vi "PS_CMD.vi"(4 "?":T1=enum."Cond_EIS", 5 "MSP_I-Range":string="C", 6 "wait until completion? (T)":bool=TRUE, 7 "GUID":string) -> (1 "File Path Out":path[](array[path]), 3 "Enum":T1=enum."Cond_EIS")   [LabVIEW 2019]
uses:
  5_Controls/PS_CMD_type-def.ctl
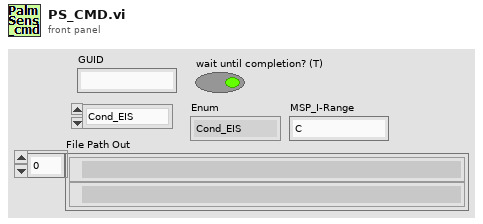
[diagram p1: front panel]
types:
  T1 = typedef "PS_CMD_type-def.ctl" = enum16{"Cond+Temp", "Cond_EIS", "Temp_EIS", "Vwind_MSP", "LongCond", "Cell1_EIS", "Cell2_EIS", "Cell3_EIS"}
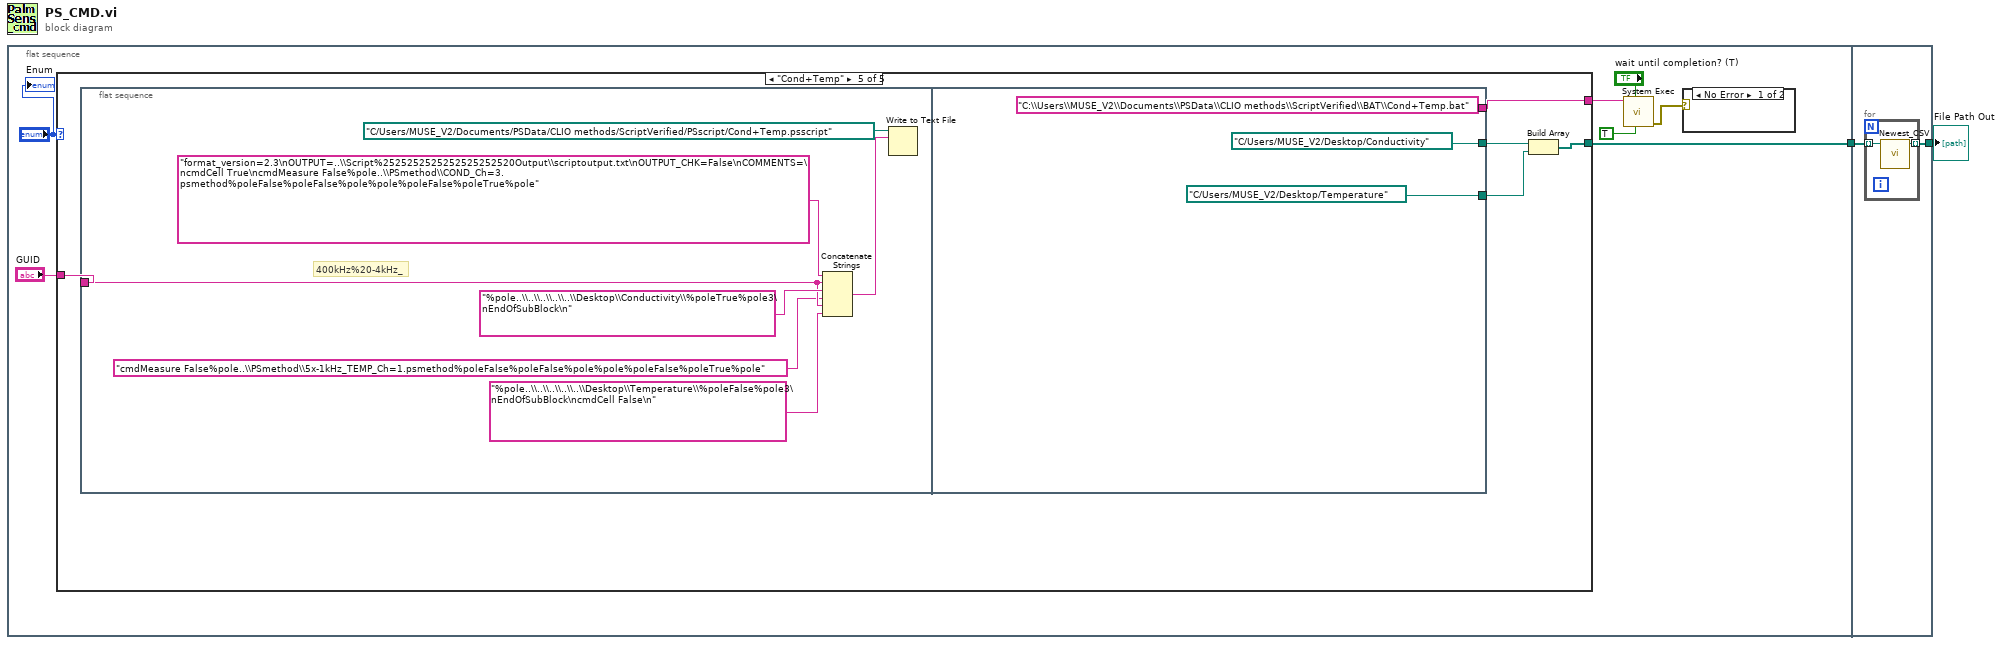
[diagram p0: block diagram]
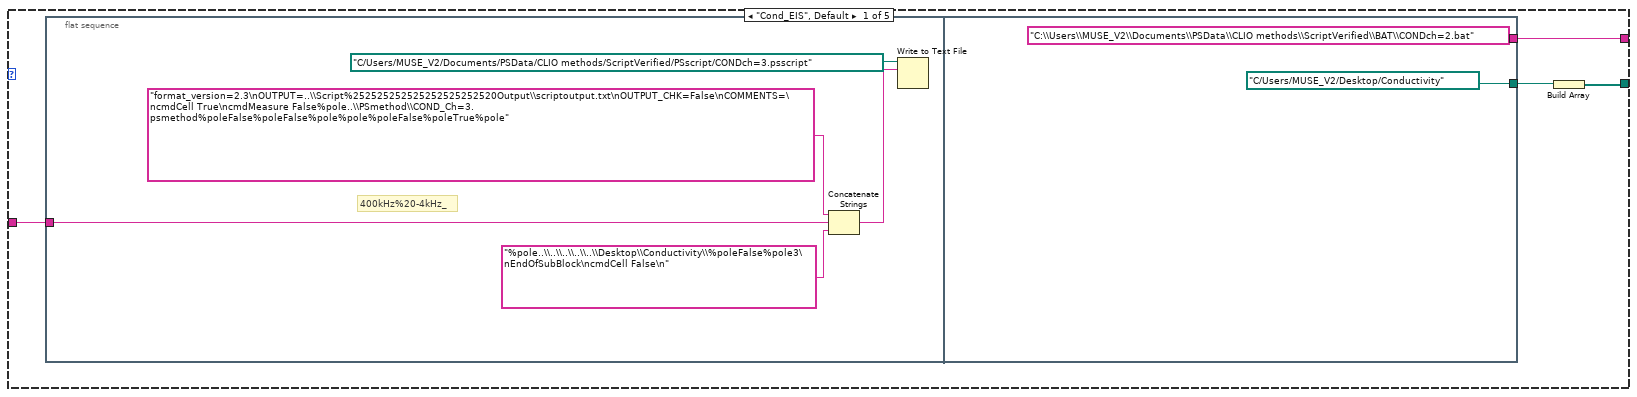
[diagram p3: hidden frame]
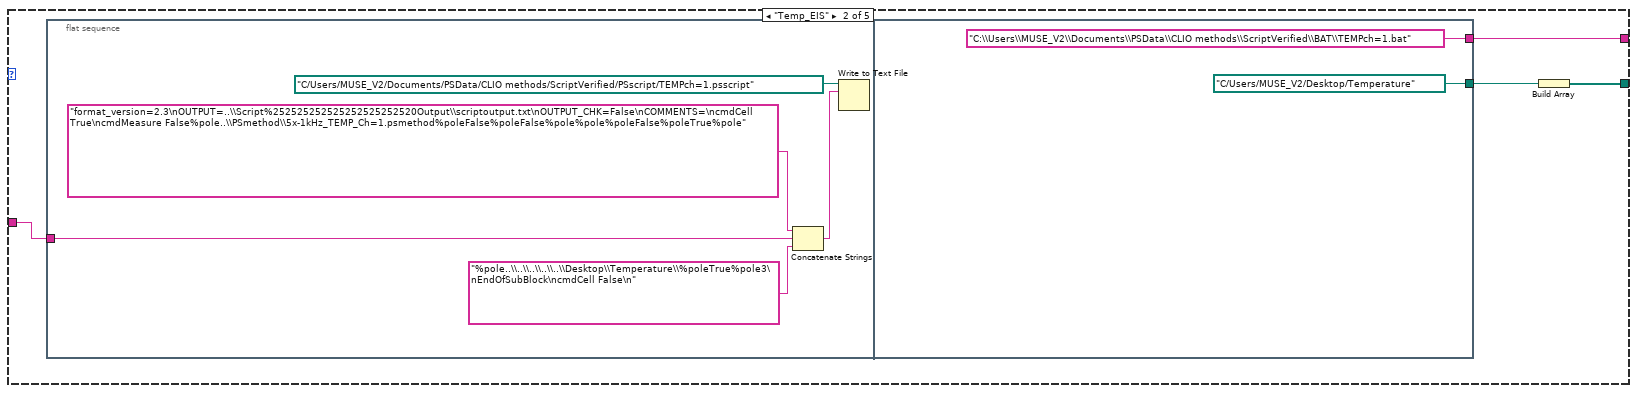
[diagram p4: hidden frame]
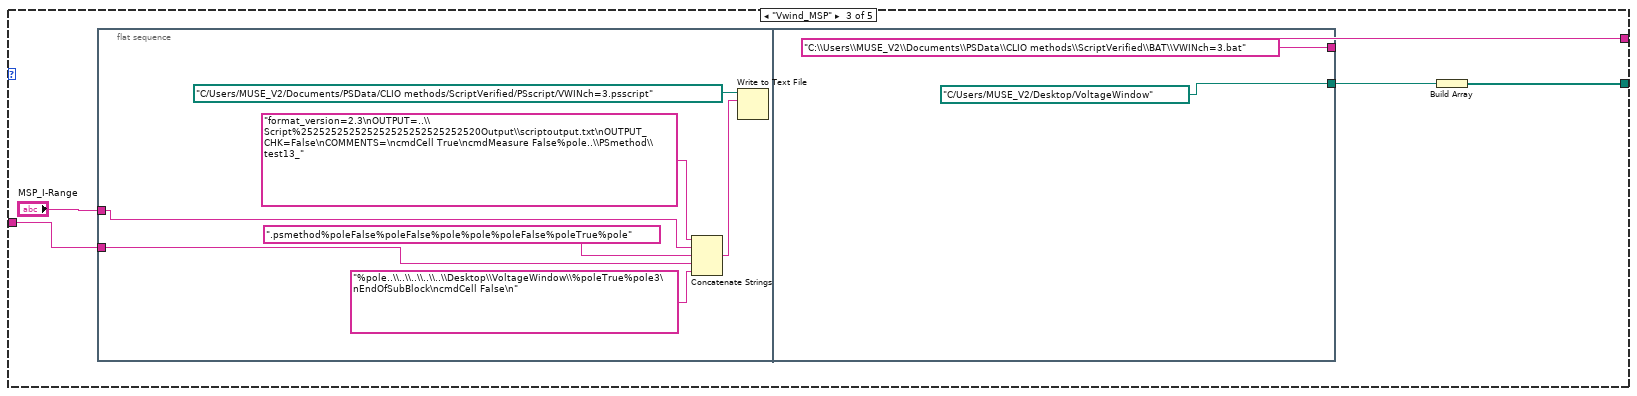
[diagram p5: hidden frame]
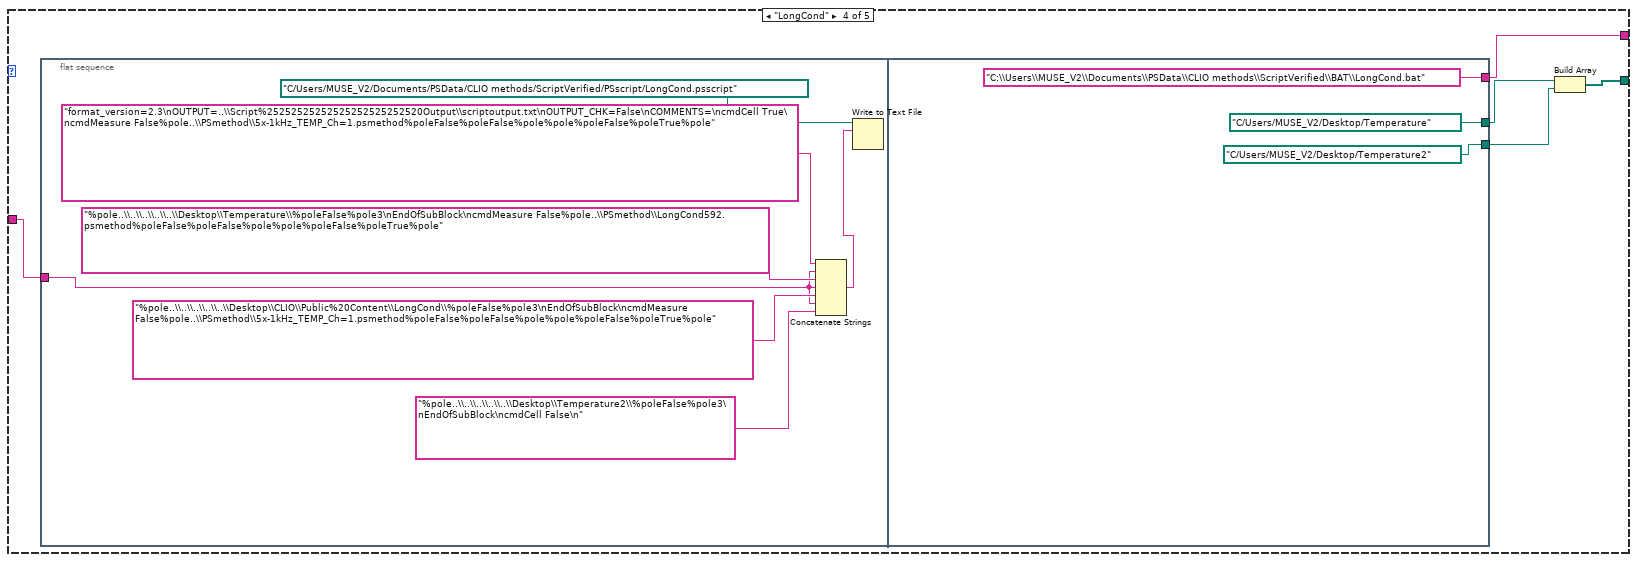
[diagram p6: hidden frame]
diagram:
  n1 = flat-sequence {
    tunnel: [w6] -> w2
    tunnel: w2 -> [w77]
    tunnel: [w76] -> w1
    frame #0 {
      n2 = case shown="\"Cond+Temp\"" "?" {
        tunnel: [w13 w24 w35 w48 w64] -> w7
        tunnel: [w10 w21 w33 w49 w62] -> w6
        tunnel: "GUID" -> [w12 w23 w36 w47 w65]
        frame "Cond_EIS", Default {
          n3 = flat-sequence {
            tunnel: w12 -> [w14]
            tunnel: ["C:\\Users\\MUSE_V2\\Documents\\PSData\\CLIO methods\\ScriptVerified\\BAT\\CONDch=2.bat" ("command line")] -> w13
            tunnel: [path "C:/Users/MUSE_V2/Desktop/Conductivity" ("Folder Path In")] -> w11
            frame #0 {
              # "400kHz%20-4kHz_"
              n4 = Concatenate Strings("format_version=2.3\nOUTPUT=..\\Script%252525252525252525252520Output\\scriptoutput.txt\nOUTPUT_CHK=False\nCOMMENTS=\ncmdCell True\ncmdMeasure False%pole..\\PSmethod\\COND_Ch=3.psmethod%poleFalse%poleFalse%pole%pole%poleFalse%poleTrue%pole" ("text"), w14, "%pole..\\..\\..\\..\\..\\Desktop\\Conductivity\\%poleFalse%pole3\nEndOfSubBlock\ncmdCell False\n" ("string")) -> (w15:string)
              n5 = Write to Text File(file (use dialog)=path "C:/Users/MUSE_V2/Documents/PSData/CLIO methods/ScriptVerified/PSscript/CONDch=3.psscript", text=w15) -> ()  [unwired: 2 in, 3 out]
            }
            frame #1 {
            }
          }
          n6 = Build Array(w11) -> (w10:path[])
        }
        frame "Temp_EIS" {
          n7 = flat-sequence {
            tunnel: w23 -> [w25]
            tunnel: ["C:\\Users\\MUSE_V2\\Documents\\PSData\\CLIO methods\\ScriptVerified\\BAT\\TEMPch=1.bat" ("command line")] -> w24
            tunnel: [path "C:/Users/MUSE_V2/Desktop/Temperature" ("Folder Path In")] -> w22
            frame #0 {
              n8 = Concatenate Strings("format_version=2.3\nOUTPUT=..\\Script%252525252525252525252520Output\\scriptoutput.txt\nOUTPUT_CHK=False\nCOMMENTS=\ncmdCell True\ncmdMeasure False%pole..\\PSmethod\\5x-1kHz_TEMP_Ch=1.psmethod%poleFalse%poleFalse%pole%pole%poleFalse%poleTrue%pole" ("text"), w25, "%pole..\\..\\..\\..\\..\\Desktop\\Temperature\\%poleTrue%pole3\nEndOfSubBlock\ncmdCell False\n" ("string")) -> (w29:string)
              n9 = Write to Text File(file (use dialog)=path "C:/Users/MUSE_V2/Documents/PSData/CLIO methods/ScriptVerified/PSscript/TEMPch=1.psscript", text=w29) -> ()  [unwired: 2 in, 3 out]
            }
            frame #1 {
            }
          }
          n10 = Build Array(w22) -> (w21:path[])
        }
        frame "Vwind_MSP" {
          n11 = flat-sequence {
            tunnel: w36 -> [w39]
            tunnel: "MSP_I-Range" -> [w37]
            tunnel: ["C:\\Users\\MUSE_V2\\Documents\\PSData\\CLIO methods\\ScriptVerified\\BAT\\VWINch=3.bat" ("command line")] -> w35
            tunnel: [path "C:/Users/MUSE_V2/Desktop/VoltageWindow" ("Folder Path In")] -> w34
            frame #0 {
              n12 = Concatenate Strings("format_version=2.3\nOUTPUT=..\\Script%252525252525252525252525252520Output\\scriptoutput.txt\nOUTPUT_CHK=False\nCOMMENTS=\ncmdCell True\ncmdMeasure False%pole..\\PSmethod\\test13_" ("text"), w37, ".psmethod%poleFalse%poleFalse%pole%pole%poleFalse%poleTrue%pole" ("string"), w39, "%pole..\\..\\..\\..\\..\\Desktop\\VoltageWindow\\%poleTrue%pole3\nEndOfSubBlock\ncmdCell False\n" ("string")) -> (w43:string)
              n13 = Write to Text File(file (use dialog)=path "C:/Users/MUSE_V2/Documents/PSData/CLIO methods/ScriptVerified/PSscript/VWINch=3.psscript", text=w43) -> ()  [unwired: 2 in, 3 out]
            }
            frame #1 {
            }
          }
          n14 = Build Array(w34) -> (w33:path[])
        }
        frame "LongCond" {
          n15 = flat-sequence {
            tunnel: w47 -> [w51]
            tunnel: ["C:\\Users\\MUSE_V2\\Documents\\PSData\\CLIO methods\\ScriptVerified\\BAT\\LongCond.bat" ("command line")] -> w48
            tunnel: [path "C:/Users/MUSE_V2/Desktop/Temperature" ("Folder Path In")] -> w50
            tunnel: [path "C:/Users/MUSE_V2/Desktop/Temperature2" ("Folder Path In")] -> w46
            frame #0 {
              # "400kHz%20-4kHz_"
              n16 = Concatenate Strings("format_version=2.3\nOUTPUT=..\\Script%25252525252525252525252520Output\\scriptoutput.txt\nOUTPUT_CHK=False\nCOMMENTS=\ncmdCell True\ncmdMeasure False%pole..\\PSmethod\\5x-1kHz_TEMP_Ch=1.psmethod%poleFalse%poleFalse%pole%pole%poleFalse%poleTrue%pole" ("text"), w51, "%pole..\\..\\..\\..\\..\\Desktop\\Temperature\\%poleFalse%pole3\nEndOfSubBlock\ncmdMeasure False%pole..\\PSmethod\\LongCond592.psmethod%poleFalse%poleFalse%pole%pole%poleFalse%poleTrue%pole" ("string"), w51, "%pole..\\..\\..\\..\\..\\Desktop\\CLIO\\Public%20Content\\LongCond\\%poleFalse%pole3\nEndOfSubBlock\ncmdMeasure False%pole..\\PSmethod\\5x-1kHz_TEMP_Ch=1.psmethod%poleFalse%poleFalse%pole%pole%poleFalse%poleTrue%pole" ("string"), w51, "%pole..\\..\\..\\..\\..\\Desktop\\Temperature2\\%poleFalse%pole3\nEndOfSubBlock\ncmdCell False\n" ("string")) -> (w54:string)
              n17 = Write to Text File(file (use dialog)=path "C:/Users/MUSE_V2/Documents/PSData/CLIO methods/ScriptVerified/PSscript/LongCond.psscript", text=w54) -> ()  [unwired: 2 in, 3 out]
            }
            frame #1 {
            }
          }
          n18 = Build Array(w50, w46) -> (w49:path[])
        }
        frame "Cond+Temp" {
          n19 = flat-sequence {
            tunnel: w65 -> [w68]
            tunnel: ["C:\\Users\\MUSE_V2\\Documents\\PSData\\CLIO methods\\ScriptVerified\\BAT\\Cond+Temp.bat" ("command line")] -> w64
            tunnel: [path "C:/Users/MUSE_V2/Desktop/Conductivity" ("Folder Path In")] -> w63
            tunnel: [path "C:/Users/MUSE_V2/Desktop/Temperature" ("Folder Path In")] -> w61
            frame #0 {
              # "400kHz%20-4kHz_"
              n20 = Concatenate Strings("format_version=2.3\nOUTPUT=..\\Script%2525252525252525252520Output\\scriptoutput.txt\nOUTPUT_CHK=False\nCOMMENTS=\ncmdCell True\ncmdMeasure False%pole..\\PSmethod\\COND_Ch=3.psmethod%poleFalse%poleFalse%pole%pole%poleFalse%poleTrue%pole" ("text"), w68, "%pole..\\..\\..\\..\\..\\Desktop\\Conductivity\\%poleTrue%pole3\nEndOfSubBlock\n" ("string"), "cmdMeasure False%pole..\\PSmethod\\5x-1kHz_TEMP_Ch=1.psmethod%poleFalse%poleFalse%pole%pole%poleFalse%poleTrue%pole" ("string"), w68, "%pole..\\..\\..\\..\\..\\Desktop\\Temperature\\%poleFalse%pole3\nEndOfSubBlock\ncmdCell False\n" ("string")) -> (w69:string)
              n21 = Write to Text File(file (use dialog)=path "C:/Users/MUSE_V2/Documents/PSData/CLIO methods/ScriptVerified/PSscript/Cond+Temp.psscript", text=w69) -> ()  [unwired: 2 in, 3 out]
            }
            frame #1 {
            }
          }
          n22 = Build Array(w63, w61) -> (w62:path[])
        }
      }
      n23 = call <vilib>:"System Exec.vi"("run minimized? (F)"=TRUE, "wait until completion? (T)"="wait until completion? (T)", "command line"=w7) -> ("error out"=w3:errorcluster)  [unwired: 5 in, 3 out]
      n24 = case shown="No Error" w3 {
        frame No Error {
        }
        frame Error {
        }
      }
      "Enum" <- "?"
    }
    frame #1 {
      n25 = for {
        tunnel: w77 -> [w79] mode=indexing
        tunnel: [w78] -> w76 mode=indexing
        n26 = call "Newest_CSV.vi"("Folder Path In"=w79) -> ("File Path Out"=w78:path)  [unwired: 9 in, 1 out]
      }
    }
  }
  "File Path Out" <- w1
